vi "Time Estimate.vi"(8 "error in (no error)":errorcluster, 9 "expmode":i32, 10 "scantype":T1(ring), 11 "Scanner.lvclass":refnum<class "Scanner.lvclass">) -> (0 "error out":errorcluster, 1 "Time Estimate":string, 2 "time":dbl[unit], 3 "Scanner.lvclass out":refnum<class "Scanner.lvclass">)   [LabVIEW 2017, in "Scanner.lvclass"]
doc: "(Dynamic) Return an estimate of the time remaining to scan over this Scanner's preconfigured Range."
uses:
  Scanner.lvclass
  Global/Set Up.vi
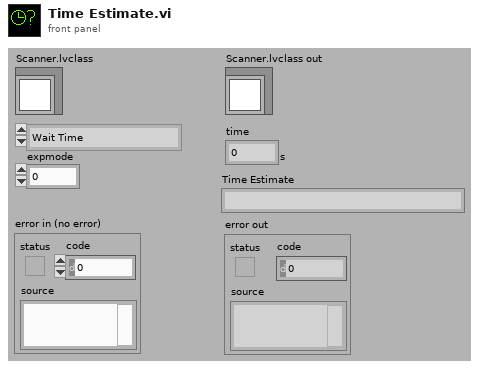
[diagram p1: front panel]
types:
  T1 = enum16{"Wait Time", "Pulse Width", "Wavelength", "Magnetic Field", "rf Scan"}
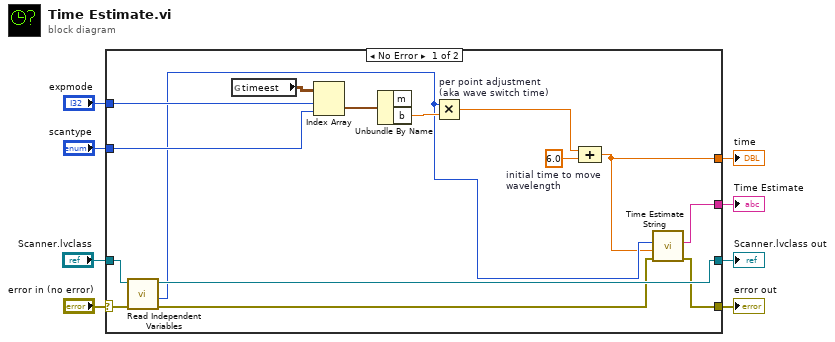
[diagram p0: block diagram]
diagram:
  n1 = case shown="No Error" "error in (no error)" {
    selector: "error in (no error)" -> [w16 w24]
    tunnel: [w11 _] -> w1
    tunnel: "expmode" -> [w22 _]
    tunnel: "scantype" -> [w17 _]
    tunnel: [w12 _] -> w6
    tunnel: [w18 w25] -> w4
    tunnel: "Scanner.lvclass" -> [w19 w25]
    tunnel: [w10 w24] -> w3
    frame No Error {
      w15 = dbl[unit] 6.0  # initial time to move wavelength
      n2 = call-dynamic "Read Independent Variables.vi"("error in (no error)"=w16, "Scanner.lvclass in"=w19) -> ("error out"=w9:errorcluster, "size"=w13:i32, "Scanner.lvclass out"=w18:refnum<class "Scanner.lvclass">)  [unwired: 7 out]
      n3 = global read "Set Up.vi" "timeest"() -> (w23:cluster{"m":dbl, "b":dbl[unit]}[][])
      n4 = Index Array(array=w23, index (row)=w22, index (col)=w17) -> (element=w21:cluster{"m":dbl, "b":dbl[unit]})
      n5 = Unbundle By Name(w21) -> ("b"=w20:dbl[unit])  [unwired: 1 out]
      n6 = Multiply "per point adjustment\n(aka wave switch time)"(x=w13, y=w20) -> (x*y=w14:dbl[unit])
      n7 = Compound Arithmetic op=ADD(w14, w15) -> (w12:dbl[unit])
      n8 = call "Time Estimate String.vi"("error in (no error)"=w9, "Time"=w12, "Steps"=w13) -> ("error out"=w10:errorcluster, "Time Estimate String"=w11:string)  [unwired: 7 in]
    }
    frame Error {
    }
  }
  "time" <- w6
  "Scanner.lvclass out" <- w4
  "error out" <- w3
  "Time Estimate" <- w1
